vi "RestoreState.vi"(8 "error in (no error)":errorcluster, 10 "State":T1, 11 "TreeControl in":refnum<vi>) -> (0 "error out":errorcluster, 3 "TreeControl out":refnum<vi>)   [LabVIEW 2019, in "TreeControlLib.lvlib"]
uses:
  TreeControlLib.lvlib
  <vilib>/Utility/Data Type/NI_Data Type.lvlib
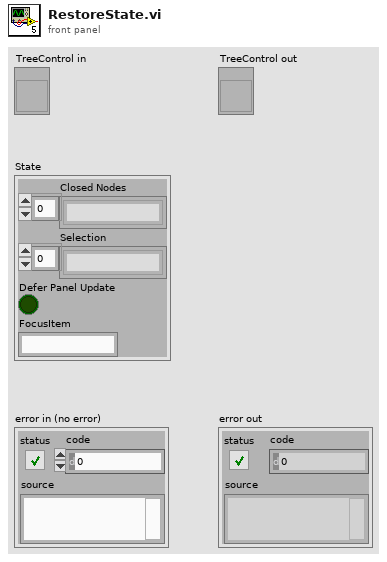
[diagram p1: front panel]
types:
  T1 = cluster{"Closed Nodes":string[], "Selection":string[], "Defer Panel Update":bool, "FocusItem":string}
  T2 = typedef "NI_Data Type.lvlib/Data Type.ctl" = enum8{"Invalid Type", "Void", "I8", "I16", "I32", "I64", "U8", "U16", "U32", "U64", "Single Float", "Double Float", "Extended Float", "Single Complex", "Double Complex", "Extended Complex", "Enum U8", "Enum U16", "Enum U32", "Enum U64", "Single Float With Unit", "Double Float With Unit", "Extended Float With Unit", "Single Complex with Unit", "Double Complex with Unit", "Extended Complex with Unit", "Boolean", "String", "Path", "Picture", "Tag", "Array", "Cluster", "Variant", "LV Variant", "Waveform", "Timestamp", "Digital Waveform", "Digital Data", "ExpressData", "Refnum", "External Data", "VI", "Poly VI", "LabVIEW Class Instance", "Fixed Point", "Set Collection", "Map Collection"}
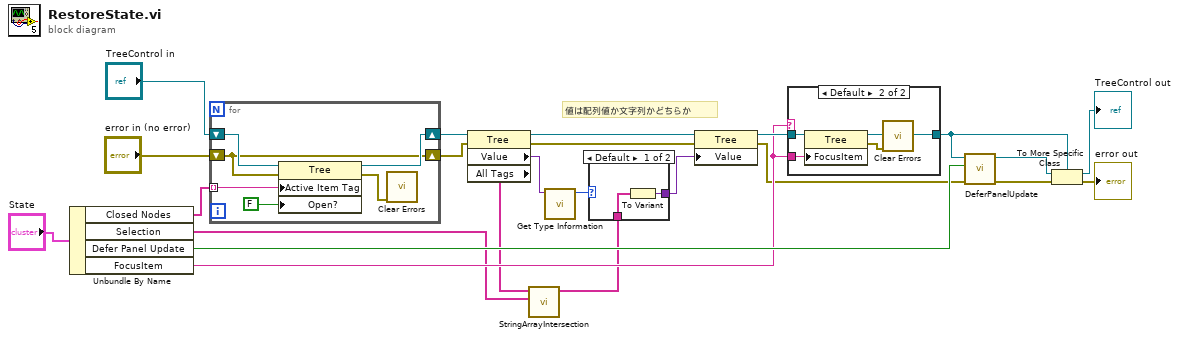
[diagram p0: block diagram]
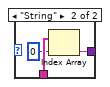
[diagram p3: hidden frame]
diagram:
  # "値は配列値か文字列かどちらか"
  n1 = Unbundle By Name("State") -> ("Closed Nodes"=w21:string[], "Selection"=w2:string[], "Defer Panel Update"=w15:bool, "FocusItem"=w7:string)
  n2 = for {
    tunnel: w21 -> [w28] mode=indexing
    shift-right: [w26] -> w14
    shift-left: "TreeControl in" -> [w27]
    shift-right: [w25] -> w6
    shift-left: "error in (no error)" -> [w25]
    n3 = property class="Tree"(reference=w27, error in=w25, "Active Item Tag"=w28, "Open?"=FALSE ("Active Item:Open?")) -> (reference out=w26:refnum<vi>, error out=w24:errorcluster)
    n4 = call <vilib>:"Clear Errors.vi"("error in (no error)"=w24) -> ()  [unwired: 5 in, 2 out]
  }
  n5 = property class="Tree"(reference=w14, error in=w6) -> (reference out=w13:refnum<vi>, error out=w5:errorcluster, "Value"=w12:variant, "All Tags"=w3:string[])
  n6 = call "StringArrayIntersection.vi"("Fewer"=w2, "More"=w3) -> ("Intersection"=w1:string[])  [unwired: 9 in]
  n7 = call <vilib>:"Get Type Information.vi"("variant"=w12) -> ("type"=w11:T2)  [unwired: 6 in, 4 out]
  n8 = case shown="Default" w11 {
    tunnel: w1 -> [w30 w34]
    tunnel: [w31 w32] -> w10
    frame Default {
      n9 = To Variant(anything=w30) -> (Variant=w31:variant)
    }
    frame "String" {
      n10 = Index Array(array=w34, index=0) -> (element=w32:string)
    }
  }
  n11 = property class="Tree"(reference=w13, error in=w5, "Value"=w10) -> (reference out=w18:refnum<vi>, error out=w4:errorcluster)
  n12 = case shown="Default" w7 {
    tunnel: w18 -> [w35 w39]
    tunnel: [w35 w38] -> w8
    tunnel: w7 -> [_ w37]
    frame "" {
    }
    frame Default {
      n13 = property class="Tree"(reference=w39, "FocusItem"=w37) -> (reference out=w38:refnum<vi>, error out=w36:errorcluster)  [unwired: 1 in]
      n14 = call <vilib>:"Clear Errors.vi"("error in (no error)"=w36) -> ()  [unwired: 5 in, 2 out]
    }
  }
  n15 = call "DeferPanelUpdate.vi"("error in (no error)"=w4, "Defer Panel Updates (T)"=w15, "Control in"=w8) -> ("error out"=w19:errorcluster, "Control out"=w16:refnum<vi>)  [unwired: 6 in, 1 out]
  n16 = To More Specific Class(target class=w8, reference=w16, error in=w19) -> (specific class reference=→"TreeControl out":refnum<vi>, error out=→"error out":errorcluster)
